vi "ZBX Set Gain ATR.vi"(7 "channel":T1, 8 "response":T2, 9 "input valid":bool, 10 "ATR state":T4, 11 "gain":u32) -> (3 "request":T3)   [LabVIEW 2023]
doc: "Change gain value for the selected ATR state and RF path. The gain value will be applied immediately. \nNote: The gain change will have immediate effect if the current ATR state is active (see DBoardState). Otherwise it will get active when the ATR state changes to the given state. \nNote: TX and Fullduplex are not the same TX states (same counts for RX and Full Duplex). One therefore needs to write both states if TX and Full Duplex (or RX and Full Duplex) are used."
uses:
  <instrlib>/niUSRP/Reference FPGA/ZBX Control/Antenna.ctl
  <instrlib>/niUSRP/Reference FPGA/ZBX Control/ZBX IO Request.ctl
  <instrlib>/niUSRP/Reference FPGA/ZBX Control/ZBX IO Response.ctl
  <instrlib>/niUSRP/Reference FPGA/ZBX Control/ATR state.ctl
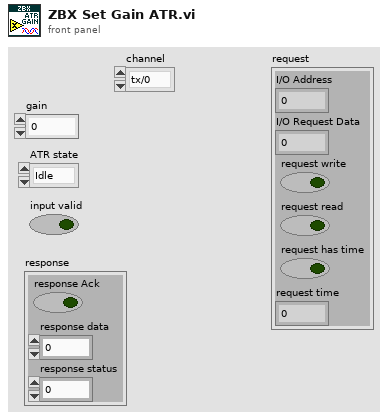
[diagram p1: front panel]
types:
  T1 = typedef "Antenna.ctl" = enum8{"tx/0", "tx/1", "rx/0", "rx/1"}
  T2 = typedef "ZBX IO Response.ctl" = cluster{"response Ack":bool, "response data":u32, "response status":fxp<+,2,2>}
  T3 = typedef "ZBX IO Request.ctl" = cluster{"I/O Address":fxp<+,20,20>, "I/O Request Data":u32, "request write":bool, "request read":bool, "request has time":bool, "request time":u64}
  T4 = typedef "ATR state.ctl" = enum8{"Idle", "RX", "TX", "TRX"}
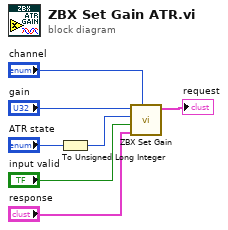
[diagram p0: block diagram]
diagram:
  n1 = To Unsigned Long Integer(number="ATR state") -> (unsigned 32bit integer=w7:u32)
  n2 = call <instrlib>:"ZBX Set Gain.vi"("channel"="channel", "response"="response", "input valid"="input valid", "config index"=w7, "gain"="gain") -> ("request"=→"request":T3)  [unwired: 5 in, 1 out]
